vi "Main.vi"() -> ()   [LabVIEW 2020, in "Multi Process.lvlib"]
uses:
  Multi Process.lvlib
panel:
  in  "stop":bool
  in  "Exe":bool
  in  "Init":bool
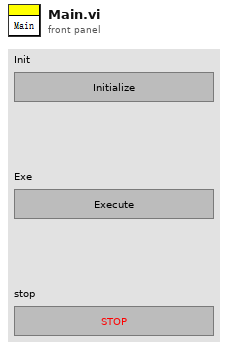
[diagram p1: front panel]
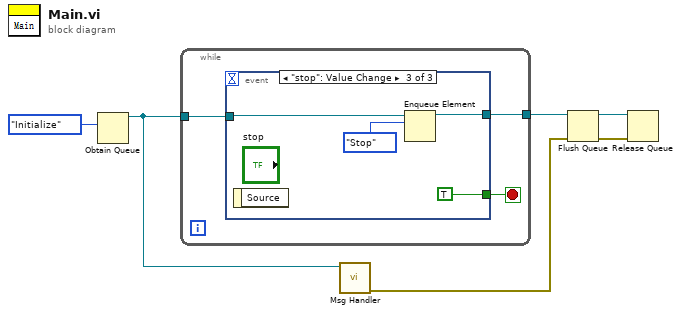
[diagram p0: block diagram]
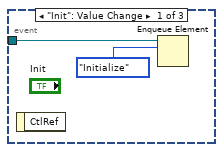
[diagram p2: hidden frame]
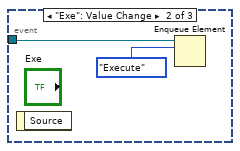
[diagram p3: hidden frame]
diagram:
  n1 = Obtain Queue(element data type=enum16{"Stop", "Execute", "Initialize"}."Initialize") -> (queue out=w2:refnum<queue>)  [unwired: 4 in, 2 out]
  n2 = while {
    tunnel: w2 -> [w9]
    tunnel: [w7] -> w4
    stop <- w8 stop-if-true
    n3 = event shown="[2] \"stop\": Value Change" {
      selector: _ -> [_ _ _]
      dyn-events: _ -> [_ _ _]
      timeout: _ -> [_ _ _]
      tunnel: w9 -> [w11 w12 w16]
      tunnel: [_ _ TRUE] -> w8
      tunnel: [_ _ w14] -> w7
      event "Init": Value Change {
        n4 = event-data() -> ()  [unwired: 1 in, 1 out]
        n5 = Enqueue Element(queue=w11, element=enum16{"Stop", "Execute", "Initialize"}."Initialize") -> ()  [unwired: 2 in, 3 out]
      }
      event "Exe": Value Change {
        n6 = event-data() -> ()  [unwired: 1 in, 1 out]
        n7 = Enqueue Element(queue=w12, element=enum16{"Stop", "Execute", "Initialize"}."Execute") -> ()  [unwired: 2 in, 3 out]
      }
      event "stop": Value Change {
        n8 = event-data() -> ()  [unwired: 1 in, 1 out]
        n9 = Enqueue Element(queue=w16, element=enum16{"Stop", "Execute", "Initialize"}."Stop") -> (queue out=w14:refnum<queue>)  [unwired: 2 in, 2 out]
      }
    }
  }
  n10 = call "Msg Handler.vi"("queue"=w2) -> ("error out"=w1:errorcluster)  [unwired: 10 in]
  n11 = Flush Queue(queue=w4, error in (no error)=w1) -> (queue out=w3:refnum<queue>, error out=w5:errorcluster)  [unwired: 1 out]
  n12 = Release Queue(queue=w3, error in (no error)=w5) -> ()  [unwired: 1 in, 3 out]
